vi "Load App.vi"(8 "error in (no error)":errorcluster, 11 "notifier":refnum<notifier>) -> (0 "error out":errorcluster)   [LabVIEW 2025, in "Config Tool.lvlib"]
doc: "Load the application into memory and start it running. The input notifier is used to send text to the splash screen to tell the user what stage the load process is in."
uses:
  Config Tool.lvlib
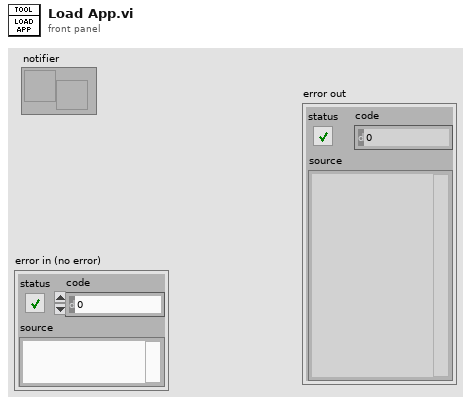
[diagram p1: front panel]
types:
  T1 = enum32{"Invalid", "Standard", "Closed", "Hidden", "Minimized", "Maximized"}
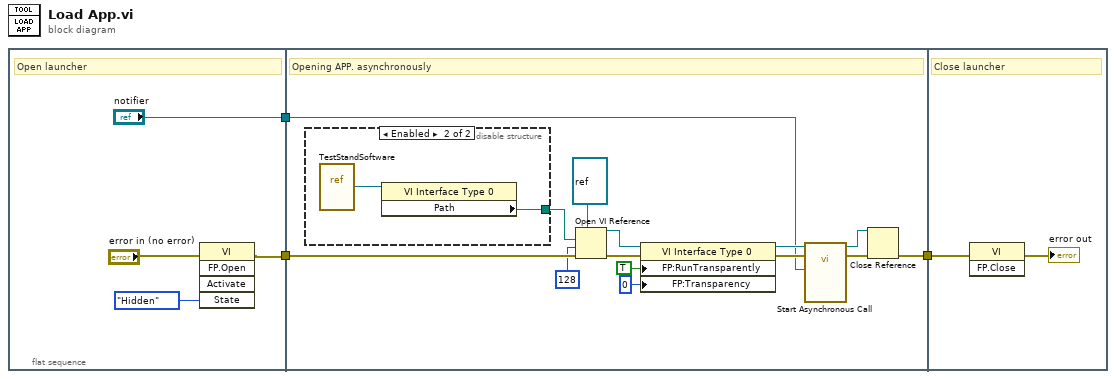
[diagram p0: block diagram]
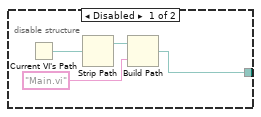
[diagram p2: hidden frame]
diagram:
  n1 = flat-sequence {
    tunnel: [w5] -> w2
    tunnel: ["notifier"] -> w1
    tunnel: [w21] -> w3
    tunnel: w2 -> [w20]
    tunnel: w1 -> [w8]
    tunnel: w3 -> [w29]
    frame #0 {
      # "Open launcher"
      n2 = invoke class="VI" method="FP.Open"(error in="error in (no error)", "State"=T1."Hidden") -> (error out=w5:errorcluster)  [unwired: 3 in, 4 out]
    }
    frame #1 {
      # "Opening APP. asynchronously"
      n3 = disable-structure shown="Enabled" {
        disable-tunnel: [w22 w27] -> w10
        frame Disabled {
          n4 = Current VI's Path() -> (path=w25:path)
          n5 = Strip Path(path=w25) -> (stripped path=w24:path)  [unwired: 1 out]
          n6 = Build Path(base path=w24, name or relative path="Main.vi") -> (appended path=w22:path)
        }
        frame Enabled {
          n7 = vi-ref "TestStandSoftware.vi"() -> (w26:refnum<vi>)
          n8 = property class="VI Interface Type 0"(reference=w26) -> ("Path"=w27:path)  [unwired: 1 in, 2 out]
        }
      }
      n9 = Open VI Reference(type specifier VI Refnum (for type only)=refnum<vi> refnum, vi path=w10, options=128, error in (no error)=w20) -> (vi reference=w18:refnum<vi>, error out=w19:errorcluster)  [unwired: 2 in]
      n10 = property class="VI Interface Type 0"(reference=w18, error in=w19, "FP:RunTransparently"=TRUE ("Front Panel Window:Run VI Transparently"), "FP:Transparency"=u8 0 ("Front Panel Window:Transparency")) -> (reference out=w13:refnum<vi>, error out=w14:errorcluster)
      n11 = call-by-ref "Start Asynchronous Call"(reference=w13, error in=w14, "notifier"=w8) -> (reference out=w12:refnum<vi>, error out=w11:errorcluster)  [unwired: 11 in]
      n12 = Close Reference(reference=w12, error in (no error)=w11) -> (error out=w21:errorcluster)
    }
    frame #2 {
      # "Close launcher"
      n13 = invoke class="VI" method="FP.Close"(error in=w29) -> (error out=→"error out":errorcluster)  [unwired: 2 in, 2 out]
    }
  }
